vi "Loop_FFT_averaged_setframes.vi"() -> ()   [LabVIEW 2021]
uses:
  <vilib>/Utility/file.llb/Write Delimited Spreadsheet (DBL).vi
  <instrlib>/Stanford Research SR78X Series/Stanford Research SR78X Series.lvlib
panel:
  out "3rd Harmonic":cluster{dbl[], dbl[]}(graph)
  out "2nd Harmonic":cluster{dbl[], dbl[]}(graph)
  out "Fundamental":cluster{dbl[], dbl[]}(graph)
  out "Frequencies of  3rd Harmonic":dbl[](array[numeric])
  out "Amplitudes of 3rd Harmonic Vpk":dbl[](array[numeric])
  out "Frequencies  of  2nd Harmonic":dbl[](array[numeric])
  out "Amplitudes of 2nd Harmonic Vpk":dbl[](array[numeric])
  out "Frequencies of fundamental":dbl[](array[numeric])
  out "Amplitudes of fundamentals":dbl[](array[numeric])
  out "Input freq in loop":dbl
  in  "Step size":dbl=1.0 min=1.0 max=10000.0
  in  "End frequency":dbl min=0.0 max=102400.0
  in  "Start frequency":dbl min=0.0 max=102400.0
  out "Bin of 3rd Harmonic":i32
  out "Bin of 2nd Harmonic":i32
  out "Amplitude of 3rd Harmonic Vpk":dbl format="%^.2e"
  out "Freq of  3rd Harmonic":dbl format="%^.2e"
  out "Amplitude of 2nd Harmonic Vpk":dbl format="%^.2e"
  out "Freq of  2nd Harmonic":dbl format="%^.2e"
  out "Amplitude of the fundamental Vpk":dbl format="%^.2e"
  out "Freq of fundamental":dbl format="%^.2e"
  out "Bin of Fundamental":i32
  in  "Waveform Function (0: Sine)":u16(ring) items=["Sine", "Square", "Pulse", "Ramp", "Noise"]
  in  "Voltage out  ( Channel 1)":u16(ring)=1 items=["Channel 1"=1, "Channel 2"=2]
  in  "Amplitude (1 Vpp)":dbl=1.0 min=0.0 max=12.0
  out "Span Hz":i32
  out "FFT":dbl[](graph)
  # "Input Signal Parameters"
  # "Data from SR 780"
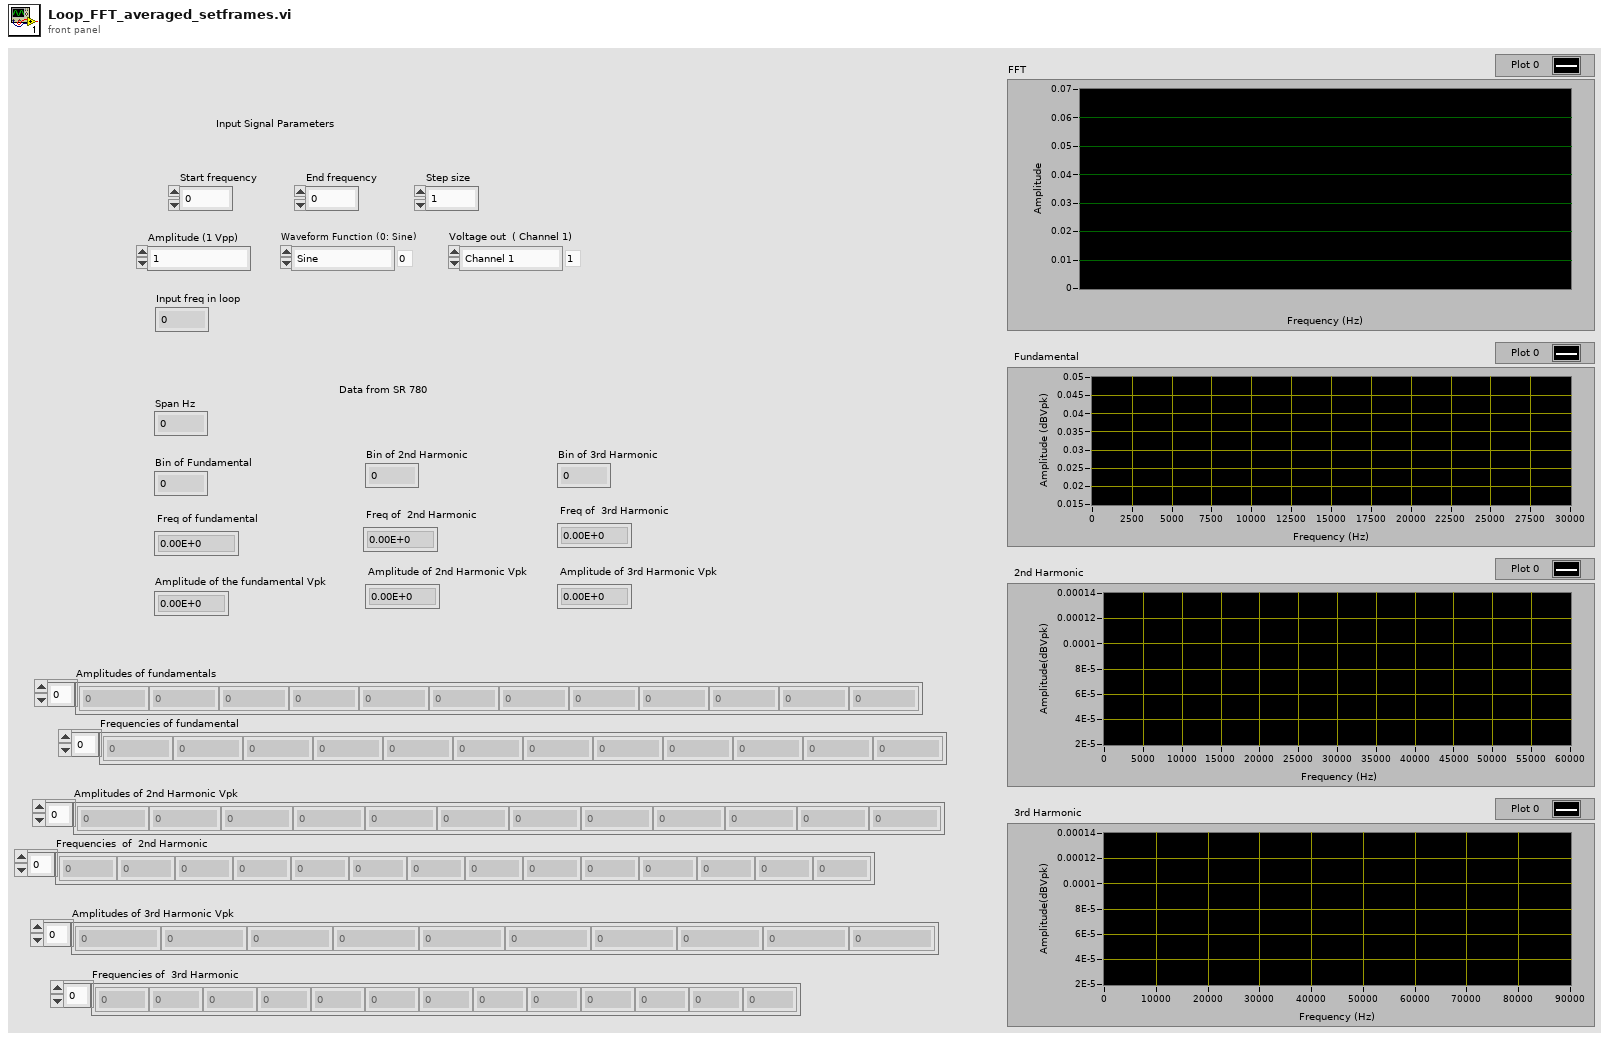
[diagram p1: front panel]
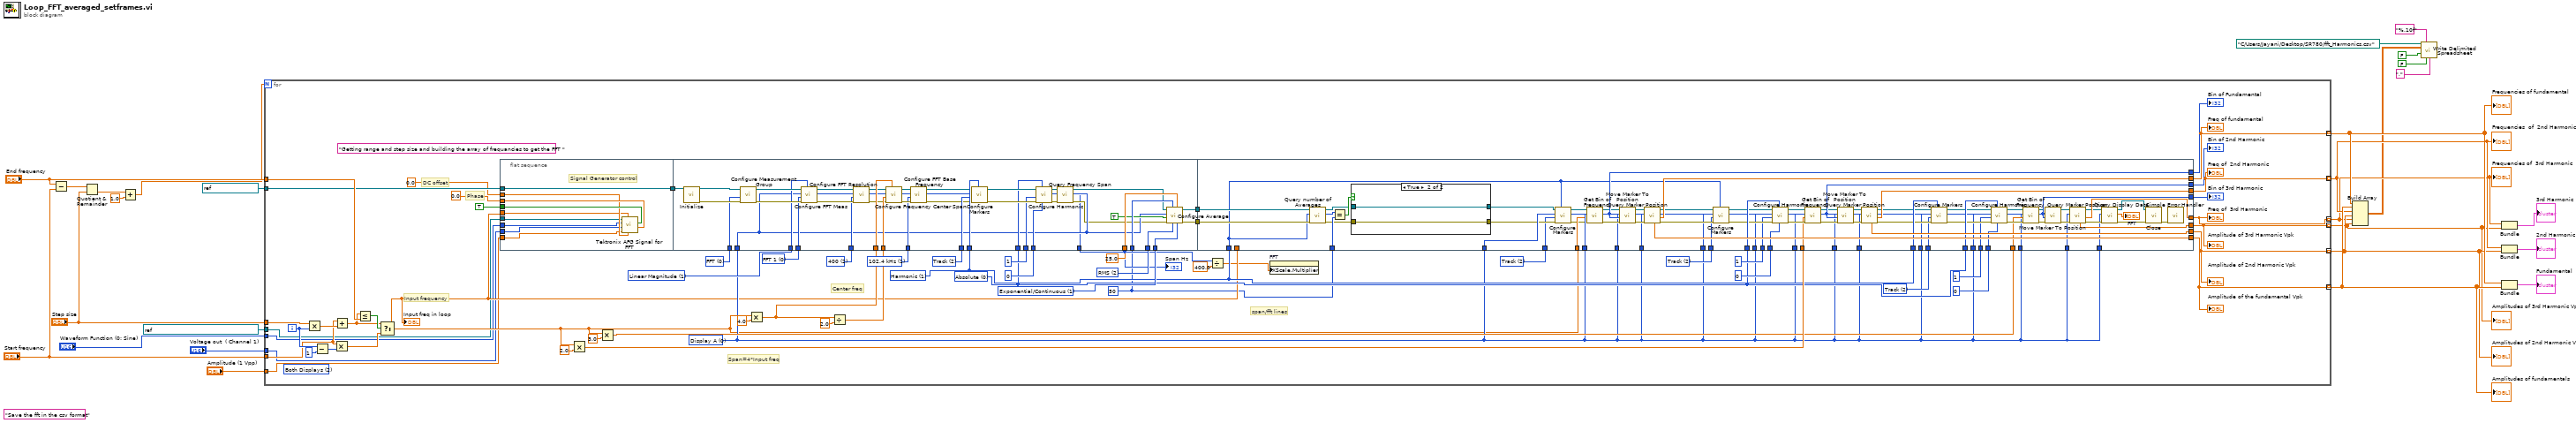
[diagram p0: block diagram]
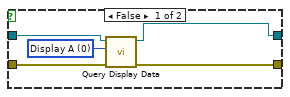
[diagram p2: hidden frame]
diagram:
  (unwired) "Save the fft in the csv format"
  n1 = Subtract(x="End frequency", y="Start frequency") -> (x-y=w22:dbl)
  n2 = Quotient & Remainder(x=w22, y="Step size") -> (floor(x/y)=w26:dbl)  [unwired: 1 out]
  n3 = Add(x=w26, y=1.0) -> (x+y=w21:dbl)
  n4 = for {
    N: w21 -> [_]
    tunnel: "Start frequency" -> [w83]
    tunnel: "Step size" -> [w90]
    tunnel: "End frequency" -> [w88]
    tunnel: "Amplitude (1 Vpp)" -> [w34]
    tunnel: "Voltage out  ( Channel 1)" -> [w33]
    tunnel: "Waveform Function (0: Sine)" -> [w32]
    tunnel: [w57] -> w6 mode=indexing
    tunnel: [w58] -> w7 mode=indexing
    tunnel: [w50] -> w4 mode=indexing
    tunnel: [w51] -> w5 mode=indexing
    tunnel: [w41] -> w2 mode=indexing
    tunnel: [w42] -> w3 mode=indexing
    tunnel: refnum<visa-resource-name> "GPIB0::0::INSTR" ("VISA resource name") -> [w66]
    tunnel: refnum<visa-resource-name> "USB0::0x0699::0x0353::2250098::INSTR" ("VISA resource name") -> [w31]
    i -> [w86]
    w30 = 2 items=["Off", "On", "Track", "Link"] ("Tracking (1: On)")
    w64 = 2 items=["None", "Vector", "RMS", "Peak Hold"] ("Average Display (0: None)")
    w65 = 1 items=["Linear/Fixed Length", "Exponential/Continuous"] ("Averaging Type (1: Exponential/Continuous)")
    w29 = 50 ("Number Of Averages (2)")
    (unwired) "Getting range and step size and building the array of frequancies to get the FFT "
    w48 = 2 items=["Off", "On", "Track", "Link"] ("Tracking (1: On)")
    w56 = 2 items=["Off", "On", "Track", "Link"] ("Tracking (1: On)")
    w46 = 0 items=["Absolute", "Relative"] ("Readout Mode (0: Absolute)")
    w49 = 1 items=["Normal", "Harmonic", "Sideband", "Band", "Frequency Damping"] ("Mode (0: Normal)")
    w74 = 2 items=["Off", "On", "Track", "Link"] ("Tracking (1: On)")
    w67 = 1 items=["100 kHz", "102.4 kHz"] ("Base Frequency (1: 102.4 kHz)")
    (unwired) 2 items=["Display A", "Display B", "Both Displays"] ("Display (2: Both Displays)")
    w68 = 2 items=["100", "200", "400", "800"] ("Resolution (2: 400)")
    w40 = 0 items=["Display A", "Display B", "Both Displays"] ("Display (2: Both Displays)")
    w70 = 0 items=["FFT 1", "FFT 2", "Power Spectrum 1", "Power Spectrum 2", "Time 1", "Time 2", "Windowed Time 1", "Windowed Time 2", "Orbit", "Coherence", "Cross Spectrum", "Frequency Response", "Capture Buffer 1", "Capture Buffer 2", "User Function 1", "User Function 2", "User Function 3", "User Function 4", "User Function 5"] ("Measurement (0: FFT 1)")
    w71 = 1 items=["Log Magnitude", "Linear Magnitude", "Magnitude Squared", "Real Part", "Imaginary Part", "Phase", "Unwrapped Phase", "Nyquist", "Nichols"] ("View (0: Log Magnitude)")
    w69 = 0 items=["FFT", "Correlation", "Octave", "Swept Sine", "Order", "Time Histogram"] ("Measurement Group (0: FFT)")
    # "Input frequency"
    # "DC offset"
    # "Phase"
    # "span/fft lines"
    # "Center freq"
    # "Span=4*Input freq"
    n5 = Multiply(x=w90, y=w86) -> (x*y=w91:dbl)
    n6 = Subtract(x=w86, y=1) -> (x-y=w84:i32)
    n7 = Multiply(x=w83, y=w84) -> (x*y=w82:dbl)
    n8 = Add(x=w83, y=w91) -> (x+y=w87:dbl)
    n9 = Less Or Equal?(x=w87, y=w88) -> (x <= y?=w89:bool)
    n10 = Select(t=w87, s=w89, f=w82) -> (s? t:f=w35:dbl)
    "Input freq in loop" <- w35
    n11 = flat-sequence {
      tunnel: w66 -> [w100]
      tunnel: [w100] -> w39
      tunnel: 0.0 ("Phase (0)") -> [w99]
      tunnel: TRUE ("Enable Output (T: Enable)") -> [w98]
      tunnel: 0.0 ("DC Offset (0.00 V)") -> [w97]
      tunnel: w35 -> [w96]
      tunnel: w34 -> [w95]
      tunnel: w33 -> [w94]
      tunnel: w32 -> [w93]
      tunnel: w31 -> [w92]
      tunnel: w81 -> [w136]
      tunnel: w80 -> [w135]
      tunnel: w46 -> [w124]
      tunnel: w49 -> [w123]
      tunnel: 0 ("Harmonic Marker (0)") -> [w122]
      tunnel: 1 ("Number Of Harmonic (1)") -> [w121]
      tunnel: w74 -> [w120]
      tunnel: w71 -> [w119]
      tunnel: w70 -> [w118]
      tunnel: w69 -> [w117]
      tunnel: w68 -> [w116]
      tunnel: w67 -> [w115]
      tunnel: w29 -> [w109]
      tunnel: w65 -> [w108]
      tunnel: w64 -> [w104]
      tunnel: 25.0 ("Time Rec Increment (100.0 %)") -> [w107]
      tunnel: [w101] -> w62
      tunnel: [w111] -> w61
      tunnel: [w110] -> w60
      tunnel: w40 -> [w105]
      tunnel: w39 -> [w114]
      tunnel: w61 -> [w151]
      tunnel: w60 -> [w150]
      tunnel: w35 -> [_]
      tunnel: w40 -> [w218]
      tunnel: [w217] -> w59
      tunnel: w35 -> [w216]
      tunnel: w40 -> [w214]
      tunnel: w40 -> [w211]
      tunnel: [w209] -> w58
      tunnel: [w208] -> w57
      tunnel: w49 -> [w149]
      tunnel: w56 -> [w206]
      tunnel: w40 -> [w205]
      tunnel: 0 ("Harmonic Marker (0)") -> [w203]
      tunnel: w46 -> [w202]
      tunnel: 1 ("Number Of Harmonic (1)") -> [w200]
      tunnel: w40 -> [w199]
      tunnel: w53 -> [w196]
      tunnel: w40 -> [w195]
      tunnel: [w193] -> w52
      tunnel: w40 -> [w191]
      tunnel: w40 -> [w188]
      tunnel: [w186] -> w51
      tunnel: [w185] -> w50
      tunnel: w49 -> [w184]
      tunnel: w48 -> [w182]
      tunnel: w40 -> [w181]
      tunnel: 0 ("Harmonic Marker (0)") -> [w179]
      tunnel: w46 -> [w178]
      tunnel: 1 ("Number Of Harmonic (1)") -> [w176]
      tunnel: w40 -> [w175]
      tunnel: w44 -> [w172]
      tunnel: w40 -> [w171]
      tunnel: [w169] -> w43
      tunnel: w40 -> [w152]
      tunnel: w40 -> [w165]
      tunnel: [w163] -> w42
      tunnel: [w162] -> w41
      tunnel: w40 -> [w156]
      tunnel: w30 -> [w141]
      tunnel: w29 -> [w147]
      frame #0 {
        # "Signal Generator control"
        n12 = call "Tektronix AFG Signal for FFT.vi"("Phase (0)"=w99, "Enable Output (T: Enable)"=w98, "DC Offset (0.00 V)"=w97, "Frequency (1000 Hz)"=w96, "Amplitude (1 Vpp)"=w95, "Channel (1 Channel 1)"=w94, "Waveform Function (0: Sine)"=w93, "VISA resource name"=w92) -> ()  [unwired: 4 in]
      }
      frame #1 {
        n13 = call <instrlib>:"Initialize.vi"("VISA resource name"=w114) -> ("VISA resource name out"=w125:refnum<visa-resource-name>, "error out"=w128:errorcluster)  [unwired: 13 in]
        n14 = call <instrlib>:"Configure Measurement Group.vi"("error in (no error)"=w128, "Measurement Group (0: FFT)"=w117, "VISA resource name"=w125) -> ("error out"=w127:errorcluster, "VISA resource name out"=w126:refnum<visa-resource-name>)  [unwired: 7 in]
        n15 = call <instrlib>:"Configure FFT Meas.vi"("View (0: Log Magnitude)"=w119, "error in (no error)"=w127, "Measurement (0: FFT 1)"=w118, "Display (2: Both Displays)"=w105, "VISA resource name"=w126) -> ("error out"=w130:errorcluster, "VISA resource name out"=w129:refnum<visa-resource-name>)  [unwired: 5 in]
        n16 = call <instrlib>:"Configure FFT Resolution.vi"("error in (no error)"=w130, "Resolution (2: 400)"=w116, "Display (2: Both Displays)"=w105, "VISA resource name"=w129) -> ("error out"=w132:errorcluster, "VISA resource name out"=w131:refnum<visa-resource-name>)  [unwired: 6 in]
        n17 = call <instrlib>:"Configure Frequency Center Span.vi"("Span (102.4E+3 Hz)"=w135, "error in (no error)"=w132, "Center (51.2E+3 Hz)"=w136, "VISA resource name"=w131) -> ("error out"=w134:errorcluster, "VISA resource name out"=w133:refnum<visa-resource-name>)  [unwired: 6 in]
        n18 = call <instrlib>:"Configure FFT Base Frequency.vi"("error in (no error)"=w134, "Base Frequency (1: 102.4 kHz)"=w115, "VISA resource name"=w133) -> ("error out"=w112:errorcluster, "VISA resource name out"=w113:refnum<visa-resource-name>)  [unwired: 7 in]
        n19 = call <instrlib>:"Configure Markers.vi"("Mode (0: Normal)"=w123, "error in (no error)"=w112, "Tracking (1: On)"=w120, "Display (2: Both Displays)"=w105, "VISA resource name"=w113) -> ("error out"=w138:errorcluster, "VISA resource name out"=w137:refnum<visa-resource-name>)  [unwired: 5 in]
        n20 = call <instrlib>:"Configure Harmonic.vi"("Harmonic Marker (0)"=w122, "Readout Mode (0: Absolute)"=w124, "error in (no error)"=w138, "Number Of Harmonic (1)"=w121, "Display (2: Both Displays)"=w105, "VISA resource name"=w137) -> ("error out"=w140:errorcluster, "VISA resource name out"=w139:refnum<visa-resource-name>)  [unwired: 4 in]
        n21 = call <instrlib>:"Query Frequency Span.vi"("error in (no error)"=w140, "Display (0: Display A)"=w105, "VISA resource name"=w139) -> ("error out"=w103:errorcluster, "Span"=w101:i32, "VISA resource name out"=w102:refnum<visa-resource-name>)  [unwired: 6 in]
        n22 = call <instrlib>:"Configure Average.vi"("Averaging Type (1: Exponential/Continuous)"=w108, "Time Rec Increment (100.0 %)"=w107, "Average Display (0: None)"=w104, "Number Of Averages (2)"=w109, "error in (no error)"=w103, "Computation Of Avg (T: Enable)"=TRUE, "Display (2: Both Displays)"=w105, "VISA resource name"=w102) -> ("error out"=w110:errorcluster, "VISA resource name out"=w111:refnum<visa-resource-name>)  [unwired: 2 in]
      }
      frame #2 {
        n23 = call <instrlib>:"Query number of Averages.vi"("error in (no error)"=w150, "Display (0: Display A)"=w149, "VISA resource name"=w151) -> ("error out"=w144:errorcluster, "No of averages"=w148:i32, "VISA resource name out"=w145:refnum<visa-resource-name>)  [unwired: 6 in]
        n24 = Equal?(x=w148, y=w147) -> (x = y?=w146:bool)
        n25 = case shown="True" w146 {
          tunnel: w145 -> [w223 w225]
          tunnel: w144 -> [w222 w224]
          tunnel: [w220 w225] -> w143
          tunnel: [w219 w224] -> w142
          frame False {
            w221 = 0 items=["Display A", "Display B"] ("Display (0: Display A)")
            n26 = call <instrlib>:"Query Display Data.vi"("error in (no error)"=w222, "Display (0: Display A)"=w221, "VISA resource name"=w223) -> ("error out"=w219:errorcluster, "VISA resource name out"=w220:refnum<visa-resource-name>)  [unwired: 6 in, 1 out]
          }
          frame True {
          }
        }
        n27 = call <instrlib>:"Configure Markers.vi"("Mode (0: Normal)"=w149, "error in (no error)"=w142, "Tracking (1: On)"=w141, "Display (2: Both Displays)"=w152, "VISA resource name"=w143) -> ("error out"=w153:errorcluster, "VISA resource name out"=w154:refnum<visa-resource-name>)  [unwired: 5 in]
        n28 = call <instrlib>:"Get Bin of Frequency.vi"("error in (no error)"=w153, "Frequency or Time (0.0)"=w216, "Display (0: Display A)"=w218, "VISA resource name"=w154) -> ("error out"=w215:errorcluster, "Bin"=w217:i32, "VISA resource name out"=w213:refnum<visa-resource-name>)  [unwired: 5 in]
        n29 = call <instrlib>:"Move Marker To Position.vi"("error in (no error)"=w215, "Position (0 bins)"=w217, "Display (0: Display A)"=w214, "VISA resource name"=w213) -> ("error out"=w212:errorcluster, "VISA resource name out"=w210:refnum<visa-resource-name>)  [unwired: 6 in]
        n30 = call <instrlib>:"Query Marker Position.vi"("error in (no error)"=w212, "Display (0: Display A)"=w211, "VISA resource name"=w210) -> ("error out"=w207:errorcluster, "X Value"=w209:dbl, "VISA resource name out"=w204:refnum<visa-resource-name>, "Y Value"=w208:dbl)  [unwired: 4 in, 1 out]
        n31 = call <instrlib>:"Configure Markers.vi"("Mode (0: Normal)"=w149, "error in (no error)"=w207, "Tracking (1: On)"=w206, "Display (2: Both Displays)"=w205, "VISA resource name"=w204) -> ("error out"=w201:errorcluster, "VISA resource name out"=w198:refnum<visa-resource-name>)  [unwired: 5 in]
        n32 = call <instrlib>:"Configure Harmonic.vi"("Harmonic Marker (0)"=w203, "Readout Mode (0: Absolute)"=w202, "error in (no error)"=w201, "Number Of Harmonic (1)"=w200, "Display (2: Both Displays)"=w199, "VISA resource name"=w198) -> ("error out"=w197:errorcluster, "VISA resource name out"=w194:refnum<visa-resource-name>)  [unwired: 4 in]
        n33 = call <instrlib>:"Get Bin of Frequency.vi"("error in (no error)"=w197, "Frequency or Time (0.0)"=w196, "Display (0: Display A)"=w195, "VISA resource name"=w194) -> ("error out"=w192:errorcluster, "Bin"=w193:i32, "VISA resource name out"=w190:refnum<visa-resource-name>)  [unwired: 5 in]
        n34 = call <instrlib>:"Move Marker To Position.vi"("error in (no error)"=w192, "Position (0 bins)"=w193, "Display (0: Display A)"=w191, "VISA resource name"=w190) -> ("error out"=w189:errorcluster, "VISA resource name out"=w187:refnum<visa-resource-name>)  [unwired: 6 in]
        n35 = call <instrlib>:"Query Marker Position.vi"("error in (no error)"=w189, "Display (0: Display A)"=w188, "VISA resource name"=w187) -> ("error out"=w183:errorcluster, "X Value"=w186:dbl, "VISA resource name out"=w180:refnum<visa-resource-name>, "Y Value"=w185:dbl)  [unwired: 4 in, 1 out]
        n36 = call <instrlib>:"Configure Markers.vi"("Mode (0: Normal)"=w184, "error in (no error)"=w183, "Tracking (1: On)"=w182, "Display (2: Both Displays)"=w181, "VISA resource name"=w180) -> ("error out"=w177:errorcluster, "VISA resource name out"=w174:refnum<visa-resource-name>)  [unwired: 5 in]
        n37 = call <instrlib>:"Configure Harmonic.vi"("Harmonic Marker (0)"=w179, "Readout Mode (0: Absolute)"=w178, "error in (no error)"=w177, "Number Of Harmonic (1)"=w176, "Display (2: Both Displays)"=w175, "VISA resource name"=w174) -> ("error out"=w173:errorcluster, "VISA resource name out"=w170:refnum<visa-resource-name>)  [unwired: 4 in]
        n38 = call <instrlib>:"Get Bin of Frequency.vi"("error in (no error)"=w173, "Frequency or Time (0.0)"=w172, "Display (0: Display A)"=w171, "VISA resource name"=w170) -> ("error out"=w168:errorcluster, "Bin"=w169:i32, "VISA resource name out"=w167:refnum<visa-resource-name>)  [unwired: 5 in]
        n39 = call <instrlib>:"Move Marker To Position.vi"("error in (no error)"=w168, "Position (0 bins)"=w169, "Display (0: Display A)"=w152, "VISA resource name"=w167) -> ("error out"=w166:errorcluster, "VISA resource name out"=w164:refnum<visa-resource-name>)  [unwired: 6 in]
        n40 = call <instrlib>:"Query Marker Position.vi"("error in (no error)"=w166, "Display (0: Display A)"=w165, "VISA resource name"=w164) -> ("error out"=w157:errorcluster, "X Value"=w163:dbl, "VISA resource name out"=w155:refnum<visa-resource-name>, "Y Value"=w162:dbl)  [unwired: 4 in, 1 out]
        n41 = call <instrlib>:"Query Display Data.vi"("error in (no error)"=w157, "Display (0: Display A)"=w156, "VISA resource name"=w155) -> ("error out"=w158:errorcluster, "Display Data"=→"FFT":dbl[], "VISA resource name out"=w159:refnum<visa-resource-name>)  [unwired: 6 in]
        n42 = call <instrlib>:"Close.vi"("VISA resource name"=w159, "error in (no error)"=w158) -> ("error out"=w160:errorcluster)  [unwired: 13 in]
        n43 = call <vilib>:"Simple Error Handler.vi"("error in (no error)"=w160) -> ()  [unwired: 4 in, 5 out]
      }
    }
    n44 = Multiply(x=w35, y=2.0) -> (x*y=w53:dbl)
    n45 = Multiply(x=w35, y=3.0) -> (x*y=w44:dbl)
    n46 = Multiply(x=w35, y=4.0) -> (x*y=w80:dbl)
    n47 = Divide(x=w80, y=2.0) -> (x/y=w81:dbl)
    n48 = Divide(x=w62, y=400.0) -> (x/y=w28:dbl)
    n49 = property on="FFT" class="WFGraph (strict)"("XScale.Multiplier"=w28) -> ()  [unwired: 2 in, 2 out]
    "Span Hz" <- w62
    "Bin of Fundamental" <- w59
    "Bin of 2nd Harmonic" <- w52
    "Bin of 3rd Harmonic" <- w43
    "Freq of  3rd Harmonic" <- w42
    "Amplitude of 3rd Harmonic Vpk" <- w41
    "Freq of  2nd Harmonic" <- w51
    "Amplitude of 2nd Harmonic Vpk" <- w50
    "Freq of fundamental" <- w58
    "Amplitude of the fundamental Vpk" <- w57
  }
  "Amplitudes of fundamentals" <- w6
  "Frequencies of fundamental" <- w7
  "Amplitudes of 2nd Harmonic Vpk" <- w4
  "Frequencies  of  2nd Harmonic" <- w5
  "Amplitudes of 3rd Harmonic Vpk" <- w2
  "Frequencies of  3rd Harmonic" <- w3
  n50 = Build Array(w7, w6, w5, w4, w3, w2) -> (w1:dbl[][])
  n51 = call-poly <vilib>:"Write Delimited Spreadsheet.vi"("file path (dialog if empty)"=path "C:/Users/Jayani/Desktop/SR780/fft_Harmonics.csv", "format (%.3f)"="%.10f", "2D data"=w1, "append to file? (new file:F)"=FALSE, "transpose? (no:F)"=FALSE, "delimiter (\\t)"="," ("delimiter (\\t)")) -> ()  [unwired: 8 in, 2 out]
  n52 = Bundle(w3, w2) -> (→"3rd Harmonic":cluster{dbl[], dbl[]})  [unwired: 1 in]
  n53 = Bundle(w5, w4) -> (→"2nd Harmonic":cluster{dbl[], dbl[]})  [unwired: 1 in]
  n54 = Bundle(w7, w6) -> (→"Fundamental":cluster{dbl[], dbl[]})  [unwired: 1 in]
